vi "挥发酚测量流程.vi"(11 "控制命令":u16(ring)=1 items=["启动测量"=1, "标样核查"=2, "零点核查"=3, "跨度核查"=4, "空白测试"=5, "平行样测试"=6, "加标回收"=7, "空白校准"=8, "标样校准"=9, "初始化（清洗）"=10, "停止测试"=11, "仪器重启"=12, "校时"=13, "模式设置"=14, "测量间隔设置"=15, "调试"=22, "填充管路"=30, "清洗管路"=31, "清洗反应杯"=32]) -> ()   [LabVIEW 2016, in "挥发酚.lvlib"]
panel:
  out "start":timestamp
  out "补测":bool
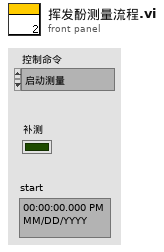
[diagram p1: front panel]
types:
  T1 = cluster{"时间标识":timestamp, "设备":string, "日志信息":string, "流程参数":string}
  T2 = cluster{"站号":u16, "量程切换":enum32{"H", "L", "AUTO"}, "控制命令":u16, "模式设置":enum16{"待机", "连续模式", "周期模式", "定点模式", "受控模式", "手动模式"}, "测量间隔":u16}
  T3 = cluster{"系统时间":timestamp, "工作状态":u16, "测量模式":enum16{"待机", "连续模式", "周期模式", "定点模式", "受控模式", "手动模式"}, "告警代码":u16, "故障代码":u16, "日志代码":u16, "软件版本":u16, "测量间隔":u16, "消解实时温度":dbl, "校准间隔（天）":u16, "校准间隔（时）":u16, "周期测量时间（23_16）":u16, "周期测量时间（15_0）":u16, "清洗周期（次数）":u16, "运行模式":u16, "自动校准状态":u16, "自动清洗状态":u16}
  T4 = cluster{"因子编码":u32, "单位":u16, "标样2参考值":sgl, "水样数据时间":timestamp, "水样实测值":sgl, "水样数据标识":string, "标样2数据时间":timestamp, "标样2实测值":sgl, "标样2数据标识":string, "空白数据时间":timestamp, "空白实测值":sgl, "空白数据标识":string, "零点核查数据时间":timestamp, "零点核查实测值":sgl, "零点核查数据标识":string, "跨度核查数据时间":timestamp, "跨度核查实测值":sgl, "跨度核查数据标识":string, "加标回收数据时间":timestamp, "加标回收实测值":sgl, "加标回收数据标识":string, "平行样数据时间":timestamp, "平行样实测值":sgl, "平行样数据标识":string, "标样1参考值":sgl, "标样1数据时间":timestamp, "标样1实测值":sgl, "标样1数据标识":string, "标样核查数据时间":timestamp, "标样核查实测值":sgl, "标样核查数据标识":string}
  T5 = cluster{"跨度值":dbl, "零点标准液浓度":dbl, "跨度标准液浓度":dbl, "标准液标准浓度":dbl, "零点标准液偏差":dbl, "跨度标准液偏差":dbl, "标准液标准偏差":dbl}
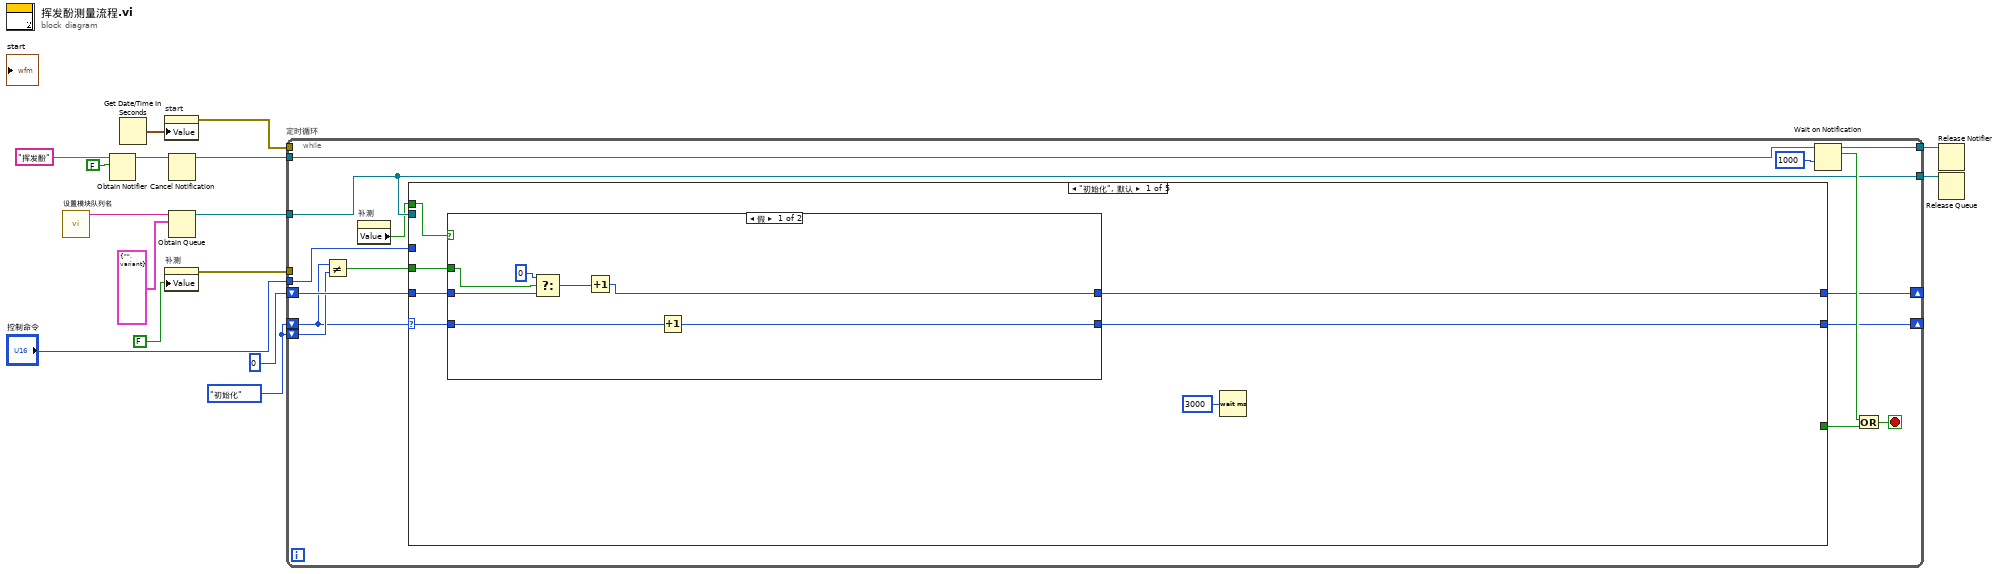
[diagram p0: block diagram]
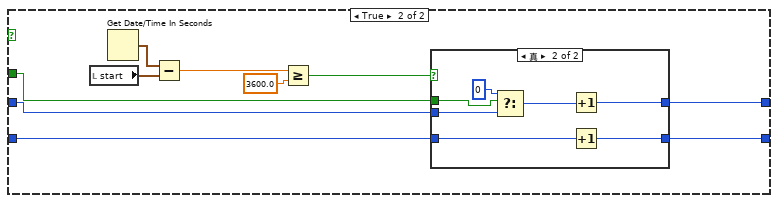
[diagram p2: hidden frame]
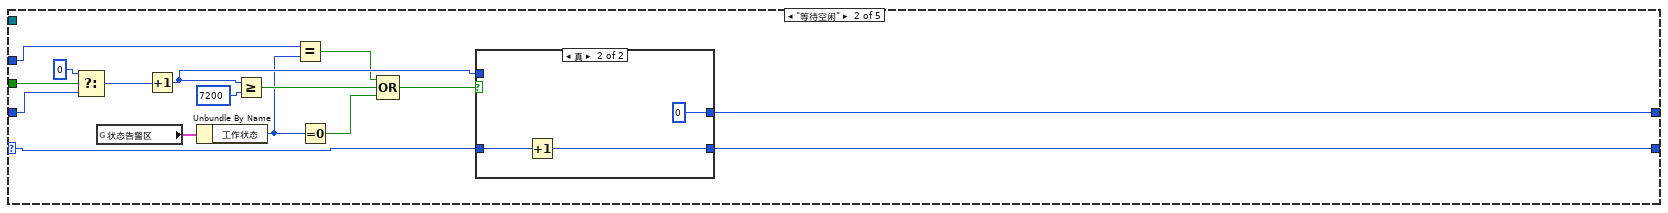
[diagram p4: hidden frame]
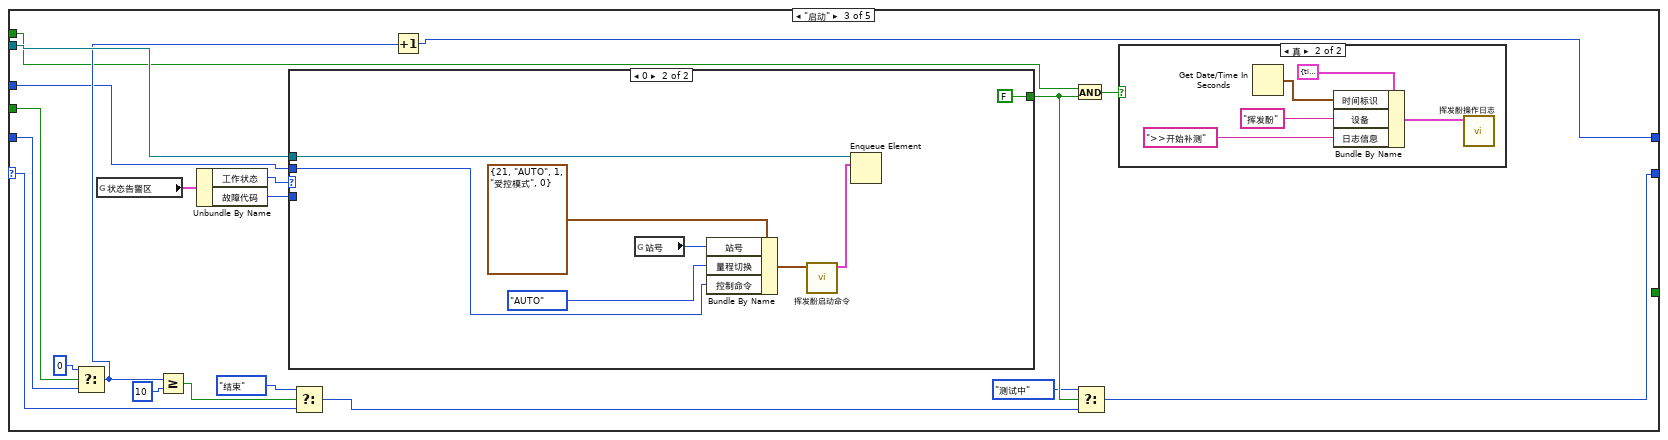
[diagram p6: hidden frame]
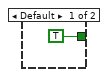
[diagram p8: hidden frame]
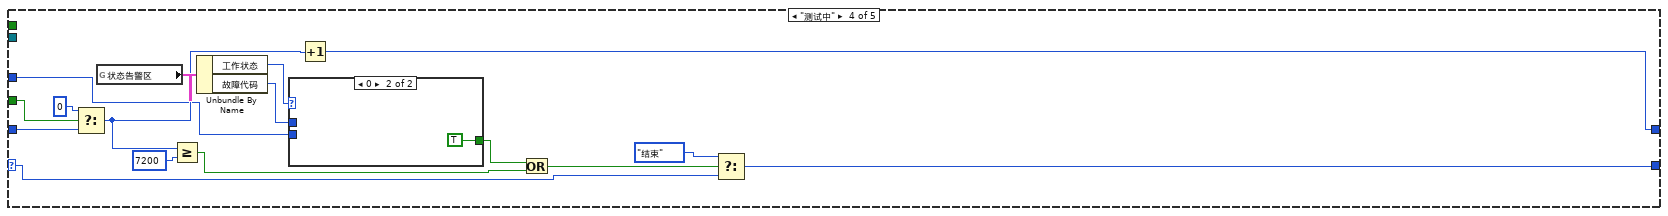
[diagram p9: hidden frame]
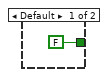
[diagram p10: hidden frame]
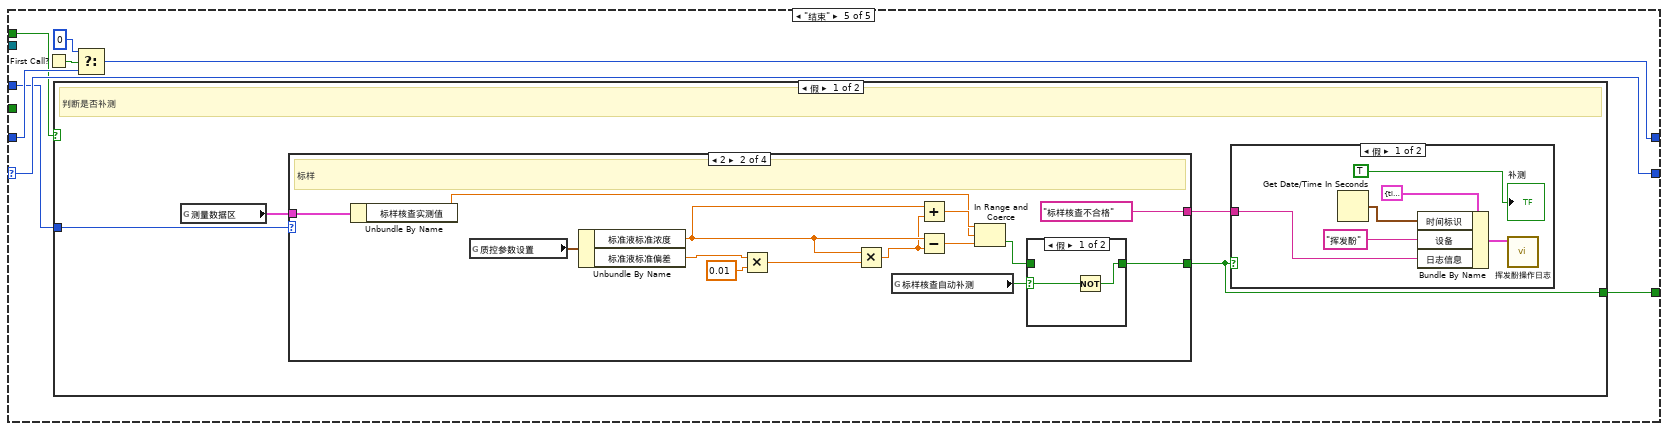
[diagram p11: hidden frame]
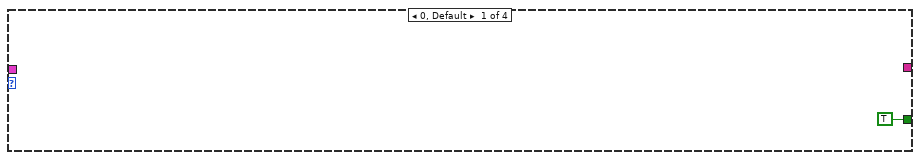
[diagram p13: hidden frame]
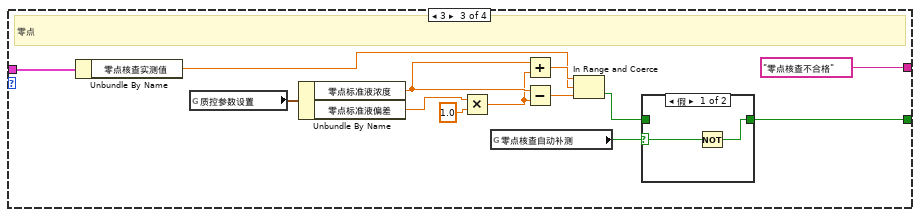
[diagram p15: hidden frame]
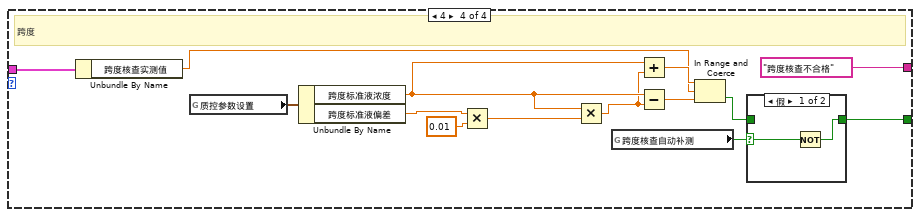
[diagram p17: hidden frame]
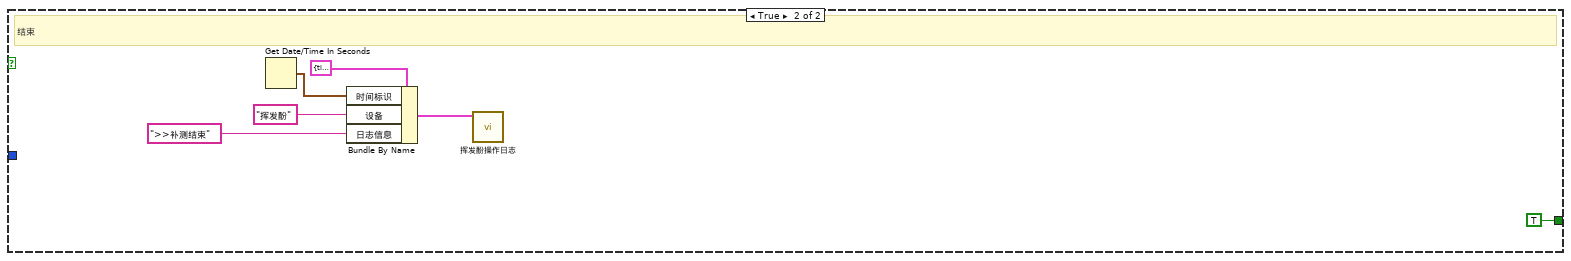
[diagram p19: hidden frame]
diagram:
  w6 = enum16{"初始化", "等待空闲", "启动", "测试中", "结束"}."初始化"
  n1 = call "设置模块队列名.vi"() -> ("Msg"=w1:string)  [unwired: 11 in]
  n2 = Obtain Notifier(name (unnamed)="挥发酚" ("名称（未命名）"), notification data type=FALSE) -> (notifier out=w12:refnum<notifier>)  [unwired: 2 in, 2 out]
  n3 = Get Date/Time In Seconds() -> (seconds since 1Jan1904=w5:timestamp)
  n4 = property on="start" class="AbsTime (严格)"("Value"=w5) -> (error out=w4:errorcluster)  [unwired: 2 in, 1 out]
  n5 = property on="补测" class="Bool (严格)"("Value"=FALSE ("补测")) -> (error out=w2:errorcluster)  [unwired: 2 in, 1 out]
  n6 = Cancel Notification(0:w12) -> (8:w11:refnum<notifier>)  [unwired: 1 in, 2 out]
  n7 = Obtain Queue(name (unnamed)=w1, element data type=cluster{"命令":string, "data":variant} {"命令"="", "data"=variant}) -> (queue out=w15:refnum<queue>)  [unwired: 3 in, 2 out]
  n8 = while "定时循环" {
    tunnel: w15 -> [w21]
    tunnel: w11 -> [w31]
    tunnel: "控制命令" -> [w27]
    shift-right: [w26] -> _
    shift-left: w6 -> [w19]
    shift-right: [w24] -> _
    shift-left: 0 -> [w25]
    tunnel: [w22] -> w8
    tunnel: [w21] -> w9
    shift-left: w6 -> [w20]
    tunnel: w4 -> [_]
    tunnel: w2 -> [_]
    stop <- w28 stop-if-true
    n9 = Not Equal?(x=w19, y=w20) -> (x != y?=w18:bool)
    n10 = property on="补测" class="Bool (严格)"() -> ("Value"=w17:bool)  [unwired: 2 in, 2 out]
    n11 = case shown="\"初始化\", 默认" w19 {
      selector: w19 -> [w38 w74 w97 w127 w145]
      tunnel: w27 -> [_ w67 w95 w122 w140]
      tunnel: w21 -> [_ _ w105 _ _]
      tunnel: [w37 w69 w91 w128 w145] -> w26
      tunnel: w25 -> [w36 w77 w101 w132 w142]
      tunnel: [w35 w68 w100 w131 w141] -> w24
      tunnel: [_ _ _ _ w138] -> w23
      tunnel: w18 -> [w34 w78 w94 w121 _]
      tunnel: w17 -> [w33 _ w89 _ w139]
      frame "初始化", Default {
        n12 = case shown="假" w33 {
          tunnel: w38 -> [w41 w55]
          tunnel: [w39 w54] -> w37
          tunnel: w36 -> [w42 w53]
          tunnel: [w40 w52] -> w35
          tunnel: w34 -> [w43 w51]
          frame False {
            n13 = Select(t=0, s=w43, f=w42) -> (s? t:f=w44:i32)
            n14 = Increment(x=w44) -> (x+1=w40:i32)
            n15 = Increment(x=w41) -> (x+1=w39:enum16{"初始化", "等待空闲", "启动", "测试中", "结束"})
          }
          frame True {
            n16 = local read "start"() -> (w49:timestamp)
            n17 = Get Date/Time In Seconds() -> (seconds since 1Jan1904=w50:timestamp)
            n18 = Subtract(x=w50, y=w49) -> (x-y=w48:dbl)
            n19 = Greater Or Equal?(x=w48, y=3600.0) -> (x >= y?=w46:bool)
            n20 = case shown="真" w46 {
              tunnel: w55 -> [w57 w64]
              tunnel: [w57 w63] -> w54
              tunnel: w53 -> [w56 w62]
              tunnel: [w56 w61] -> w52
              tunnel: w51 -> [_ w60]
              frame False {
              }
              frame True {
                n21 = Select(t=0, s=w60, f=w62) -> (s? t:f=w58:i32)
                n22 = Increment(x=w58) -> (x+1=w61:i32)
                n23 = Increment(x=w64) -> (x+1=w63:enum16{"初始化", "等待空闲", "启动", "测试中", "结束"})
              }
            }
          }
        }
        n24 = Wait (ms)(milliseconds to wait=u32 3000 ("等待时间（毫秒）")) -> ()  [unwired: 1 out]
      }
      frame "等待空闲" {
        n25 = Select(t=0, s=w78, f=w77) -> (s? t:f=w79:i32)
        n26 = global read "VAR挥发酚全局变量.vi" "状态告警区"() -> (w75:T3)
        n27 = Increment(x=w79) -> (x+1=w70:i32)
        n28 = Unbundle By Name(w75) -> ("工作状态"=w66:u16)
        n29 = Greater Or Equal?(x=w70, y=7200) -> (x >= y?=w73:bool)
        n30 = Equal?(x=w67, y=w66) -> (x = y?=w65:bool)
        n31 = Equal To 0?(x=w66) -> (x = 0?=w72:bool)
        n32 = Compound Arithmetic op=OR ("复合运算")(w65, w73, w72) -> (w71:bool)
        n33 = case shown="真" w71 {
          tunnel: w74 -> [w81 w85]
          tunnel: w70 -> [w82 _]
          tunnel: [w81 w84] -> w69
          tunnel: [w82 0] -> w68
          frame False {
          }
          frame True {
            n34 = Increment(x=w85) -> (x+1=w84:enum16{"初始化", "等待空闲", "启动", "测试中", "结束"})
          }
        }
      }
      frame "启动" {
        n35 = Select(t=0, s=w94, f=w101) -> (s? t:f=w99:i32)
        n36 = global read "VAR挥发酚全局变量.vi" "状态告警区"() -> (w104:T3)
        n37 = Greater Or Equal?(x=w99, y=10) -> (x >= y?=w92:bool)
        n38 = Unbundle By Name(w104) -> ("工作状态"=w103:u16, "故障代码"=w96:u16)
        n39 = case shown="0" w103 {
          tunnel: w95 -> [_ w118]
          tunnel: w105 -> [_ w119]
          tunnel: [TRUE FALSE] -> w90
          tunnel: w96 -> [_ _]
          frame Default {
          }
          frame 0 {
            n40 = global read "挥发酚断电保存全局变量.vi" "站号"() -> (w115:u16)
            n41 = Bundle By Name(cluster=T2 {"站号"=21, "量程切换"=enum."AUTO", "控制命令"=1, "模式设置"=enum."受控模式", "测量间隔"=0} ("参数"), "站号"=w115, "量程切换"=enum32{"H", "L", "AUTO"}."AUTO", "控制命令"=w118) -> (w112:T2)
            n42 = call "挥发酚启动命令.vi"("参数"=w112) -> ("启动命令"=w116:cluster{"命令":string, "data":variant})  [unwired: 10 in]
            n43 = Enqueue Element(queue=w119, element=w116) -> ()  [unwired: 2 in, 3 out]
          }
        }
        n44 = Select(t=enum16{"初始化", "等待空闲", "启动", "测试中", "结束"}."结束", s=w92, f=w97) -> (s? t:f=w93:enum16{"初始化", "等待空闲", "启动", "测试中", "结束"})
        n45 = Increment(x=w99) -> (x+1=w100:i32)
        n46 = And(x=w89, y=w90) -> (x .and. y?=w88:bool)
        n47 = Select(t=enum16{"初始化", "等待空闲", "启动", "测试中", "结束"}."测试中", s=w90, f=w93) -> (s? t:f=w91:enum16{"初始化", "等待空闲", "启动", "测试中", "结束"})
        n48 = case shown="真" w88 {
          frame False {
          }
          frame True {
            n49 = Get Date/Time In Seconds() -> (seconds since 1Jan1904=w108:timestamp)
            n50 = Bundle By Name(cluster=T1 {"时间标识"=timestamp(0 s since 1904-01-01), "设备"="", "日志信息"="", "流程参数"=""} ("data in"), "时间标识"=w108, "设备"="挥发酚", "日志信息"=">>开始补测") -> (w110:T1)
            n51 = call "挥发酚操作日志.vi"("data in"=w110) -> ()  [unwired: 11 in]
          }
        }
      }
      frame "测试中" {
        n52 = Select(t=0, s=w121, f=w132) -> (s? t:f=w130:i32)
        n53 = global read "VAR挥发酚全局变量.vi" "状态告警区"() -> (w135:T3)
        n54 = Greater Or Equal?(x=w130, y=7200) -> (x >= y?=w126:bool)
        n55 = Unbundle By Name(w135) -> ("工作状态"=w134:u16, "故障代码"=w123:u16)
        n56 = case shown="0" w134 {
          tunnel: w122 -> [_ _]
          tunnel: [FALSE TRUE] -> w124
          tunnel: w123 -> [_ _]
          frame Default {
          }
          frame 0 {
          }
        }
        n57 = Increment(x=w130) -> (x+1=w131:i32)
        n58 = Or(x=w124, y=w126) -> (x .or. y?=w125:bool)
        n59 = Select(t=enum16{"初始化", "等待空闲", "启动", "测试中", "结束"}."结束", s=w125, f=w127) -> (s? t:f=w128:enum16{"初始化", "等待空闲", "启动", "测试中", "结束"})
      }
      frame "结束" {
        n60 = First Call?() -> (First Call?: T/F=w144:bool)
        n61 = case shown="假" w139 {
          tunnel: w140 -> [w149 _]
          tunnel: [w146 TRUE] -> w138
          frame False {
            # "判断是否补测"
            n62 = global read "VAR挥发酚全局变量.vi" "测量数据区"() -> (w148:T4)
            n63 = case shown="2" w149 {
              tunnel: w148 -> [_ w170 w176 w195]
              tunnel: [TRUE w161 w175 w194] -> w146
              tunnel: [_ "标样核查不合格" ("日志信息") "零点核查不合格" ("日志信息") "跨度核查不合格" ("日志信息")] -> w147
              frame 0, Default {
              }
              frame 2 {
                # "标样"
                n64 = Unbundle By Name(w170) -> ("标样核查实测值"=w162:sgl)
                n65 = global read "挥发酚断电保存全局变量.vi" "质控参数设置"() -> (w163:T5)
                n66 = Unbundle By Name(w163) -> ("标准液标准浓度"=w158:dbl, "标准液标准偏差"=w165:dbl)
                n67 = Multiply(x=w165, y=0.01) -> (x*y=w159:dbl)
                n68 = Multiply(x=w158, y=w159) -> (x*y=w157:dbl)
                n69 = global read "挥发酚断电保存全局变量.vi" "标样核查自动补测"() -> (w168:bool)
                n70 = Add(x=w158, y=w157) -> (x+y=w166:dbl)
                n71 = Subtract(x=w158, y=w157) -> (x-y=w167:dbl)
                n72 = In Range and Coerce(upper limit=w166, x=w162, lower limit=w167) -> (In Range?=w169:bool)  [unwired: 1 out]
                n73 = case shown="假" w168 {
                  selector: w168 -> [w172 _]
                  tunnel: w169 -> [_ w173]
                  tunnel: [w171 w173] -> w161
                  frame False {
                    n74 = Not(x=w172) -> (.not. x?=w171:bool)
                  }
                  frame True {
                  }
                }
              }
              frame 3 {
                # "零点"
                n75 = Unbundle By Name(w176) -> ("零点核查实测值"=w177:sgl)
                n76 = global read "挥发酚断电保存全局变量.vi" "质控参数设置"() -> (w178:T5)
                n77 = Unbundle By Name(w178) -> ("零点标准液浓度"=w181:dbl, "零点标准液偏差"=w182:dbl)
                n78 = Multiply(x=w182, y=1.0) -> (x*y=w180:dbl)
                n79 = global read "挥发酚断电保存全局变量.vi" "零点核查自动补测"() -> (w185:bool)
                n80 = Add(x=w181, y=w180) -> (x+y=w183:dbl)
                n81 = Subtract(x=w181, y=w180) -> (x-y=w184:dbl)
                n82 = In Range and Coerce(upper limit=w183, x=w177, lower limit=w184) -> (In Range?=w186:bool)  [unwired: 1 out]
                n83 = case shown="假" w185 {
                  selector: w185 -> [w188 _]
                  tunnel: w186 -> [_ w189]
                  tunnel: [w187 w189] -> w175
                  frame False {
                    n84 = Not(x=w188) -> (.not. x?=w187:bool)
                  }
                  frame True {
                  }
                }
              }
              frame 4 {
                # "跨度"
                n85 = Unbundle By Name(w195) -> ("跨度核查实测值"=w196:sgl)
                n86 = global read "挥发酚断电保存全局变量.vi" "质控参数设置"() -> (w197:T5)
                n87 = Unbundle By Name(w197) -> ("跨度标准液浓度"=w191:dbl, "跨度标准液偏差"=w199:dbl)
                n88 = Multiply(x=w199, y=0.01) -> (x*y=w192:dbl)
                n89 = Multiply(x=w191, y=w192) -> (x*y=w190:dbl)
                n90 = global read "挥发酚断电保存全局变量.vi" "跨度核查自动补测"() -> (w202:bool)
                n91 = Add(x=w191, y=w190) -> (x+y=w200:dbl)
                n92 = Subtract(x=w191, y=w190) -> (x-y=w201:dbl)
                n93 = In Range and Coerce(upper limit=w200, x=w196, lower limit=w201) -> (In Range?=w203:bool)  [unwired: 1 out]
                n94 = case shown="假" w202 {
                  selector: w202 -> [w205 _]
                  tunnel: w203 -> [_ w206]
                  tunnel: [w204 w206] -> w194
                  frame False {
                    n95 = Not(x=w205) -> (.not. x?=w204:bool)
                  }
                  frame True {
                  }
                }
              }
            }
            n96 = case shown="假" w146 {
              tunnel: w147 -> [w151 _]
              frame False {
                n97 = Get Date/Time In Seconds() -> (seconds since 1Jan1904=w153:timestamp)
                n98 = Bundle By Name(cluster=T1 {"时间标识"=timestamp(0 s since 1904-01-01), "设备"="", "日志信息"="", "流程参数"=""} ("data in"), "时间标识"=w153, "设备"="挥发酚", "日志信息"=w151) -> (w152:T1)
                n99 = call "挥发酚操作日志.vi"("data in"=w152) -> ()  [unwired: 11 in]
                "补测" <- TRUE ("补测")
              }
              frame True {
              }
            }
          }
          frame True {
            # "结束"
            n100 = Get Date/Time In Seconds() -> (seconds since 1Jan1904=w209:timestamp)
            n101 = Bundle By Name(cluster=T1 {"时间标识"=timestamp(0 s since 1904-01-01), "设备"="", "日志信息"="", "流程参数"=""} ("data in"), "时间标识"=w209, "设备"="挥发酚", "日志信息"=">>补测结束") -> (w211:T1)
            n102 = call "挥发酚操作日志.vi"("data in"=w211) -> ()  [unwired: 11 in]
          }
        }
        n103 = Select(t=0, s=w144, f=w142) -> (s? t:f=w141:i32)
      }
    }
    n104 = Wait on Notification(notifier=w31, timeout in ms (-1)=1000 ("超时毫秒(-1)")) -> (notifier out=w22:refnum<notifier>, notification=w29:bool)  [unwired: 2 in, 2 out]
    n105 = Or(x=w29, y=w23) -> (x .or. y?=w28:bool)
  }
  n106 = Release Notifier(notifier=w8) -> ()  [unwired: 2 in, 3 out]
  n107 = Release Queue(queue=w9) -> ()  [unwired: 2 in, 3 out]
